vi "Parse_Return_Data.vi"(10 "String":string, 11 "data in":string) -> (1 "TCP Sent Data":string, 2 "x = y?":bool, 3 "Return Value":string, 4 "TCP Received Data":string)   [LabVIEW 2018]
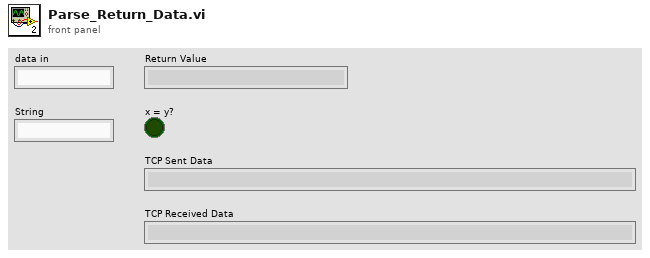
[diagram p1: front panel]
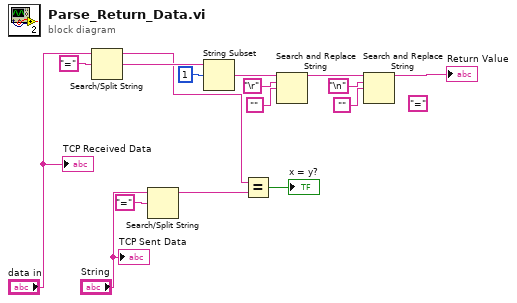
[diagram p0: block diagram]
diagram:
  (unwired) "="
  n1 = Search/Split String(string="data in", search string/char (-)="=") -> (substring before match=w15:string, match + rest of string=w16:string)  [unwired: 1 in, 1 out]
  n2 = Search/Split String(string="String", search string/char (-)="=") -> (substring before match=w13:string)  [unwired: 1 in, 2 out]
  n3 = String Subset(string=w16, offset (0)=1) -> (substring=w2:string)  [unwired: 1 in]
  n4 = Equal?(x=w15, y=w13) -> (x = y?=→"x = y?":bool)
  n5 = Search and Replace String(input string=w2, search string="\r", replace string="") -> (result string=w6:string)  [unwired: 5 in, 3 out]
  n6 = Search and Replace String(input string=w6, search string="\n", replace string="") -> (result string=→"Return Value":string)  [unwired: 5 in, 3 out]
  "TCP Received Data" <- "data in"
  "TCP Sent Data" <- "String"
